vi "CutArray.vi"(9 "Original":dbl[](array[numeric]), 10 "# to Cut":i32=4, 11 "Cut?":bool) -> (3 "result":dbl[](array[numeric]))   [LabVIEW 2013]
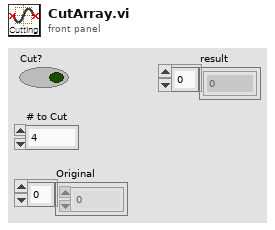
[diagram p1: front panel]
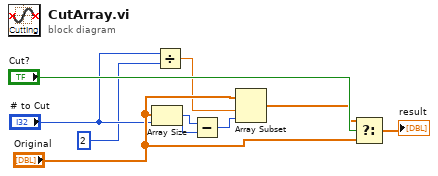
[diagram p0: block diagram]
diagram:
  n1 = Array Size(array="Original") -> (size(s)=w5:i32)
  n2 = Divide(x="# to Cut", y=2 ("index")) -> (x/y=w1:dbl)
  n3 = Subtract(x=w5, y="# to Cut") -> (x-y=w4:i32)
  n4 = Array Subset(array="Original", index=w1, length=w4) -> (w7:dbl[])
  n5 = Select(t=w7, s="Cut?", f="Original") -> (s? t:f=→"result":dbl[])
